vi "new sensor read.vi"(0 "Device Handle 2":i32, 2 "Pipe handle":i32, 3 "PixelSize":u16) -> (5 "Data buffer":u16[](array[numeric]), 6 "return type":u16, 7 "XY Graph":cluster{i32[], "Buffer":u16[]}(graph) caption="XY Glaph", 9 "appended array":u16[][](array[numeric]))   [LabVIEW 2019]
uses:
  specu1a.dll
panel:
  in  "default value":u16[](array[numeric])
  in  "default value 2":u16[](array[numeric])
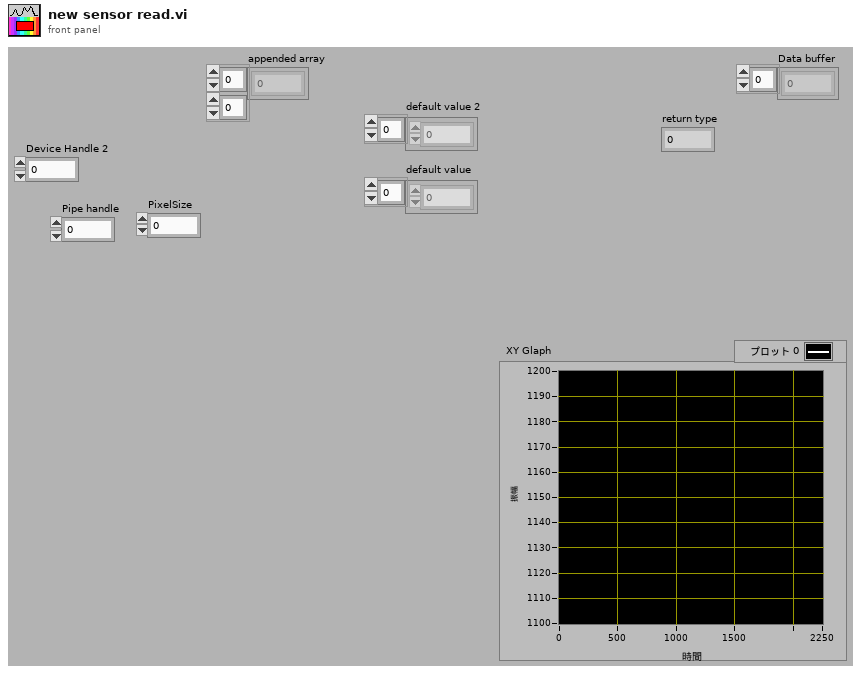
[diagram p1: front panel]
types:
  T1 = cluster{"default value 2":i32[], "Data buffer":u16[]}
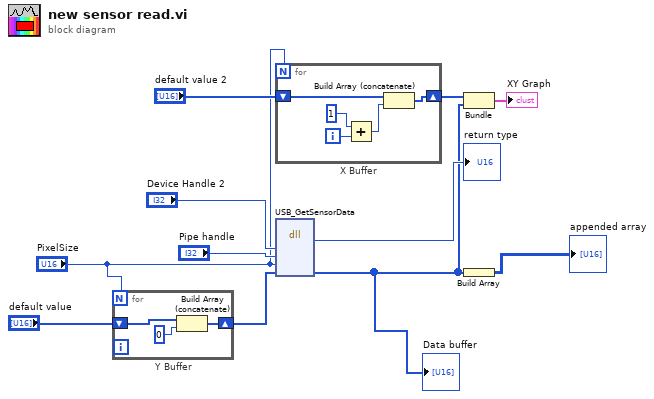
[diagram p0: block diagram]
diagram:
  n1 = for "Y Buffer" {
    N: "PixelSize" -> [_]
    shift-right: [w14] -> w6
    shift-left: "default value" -> [w13]
    n2 = Build Array (concatenate)(w13, 0) -> (w14:i32[])
  }
  n3 = for "X Buffer" {
    N: "PixelSize" -> [_]
    shift-right: [w19] -> w4
    shift-left: "default value 2" -> [w18]
    i -> [w17]
    n4 = Add(x=1, y=w17) -> (x+y=w15:i32)
    n5 = Build Array (concatenate)(w18, w15) -> (w19:i32[])
  }
  n6 = dll-call lib="C:/Users/martzlab/Desktop/SIO 179/Nitrate/64/EvaluationSoftware/minispec labview/Hamamatsu Spectrometer Dll/specu1a.dll" fn="USB_GetSensorData" label="1.0.0 Get sensor data"("Device Handle"="Device Handle 2", "Pipe handle"="Pipe handle", "Pixel size"="PixelSize", "Data buffer"=w6) -> ("return type"=→"return type":u16, "Data buffer"=w2:u16[])  [unwired: 6 in, 2 out]
  "Data buffer" <- w2
  n7 = Bundle("default value 2"=w4, "Data buffer"=w2) -> (→"XY Graph":T1)  [unwired: 1 in]
  n8 = Build Array(w2) -> (→"appended array":u16[][])
